vi "Actor Core.vi"(8 "error in (no error)":errorcluster, 11 "Operator UI.lvclass":refnum<class "Server UI.lvclass">) -> (0 "error out":errorcluster, 3 "Actor Framework.lvlib:Actor":refnum<class "Actor.lvclass">)   [LabVIEW 2026, in "Server UI.lvlib" / "Server UI.lvclass"]
doc: "This is Actor Core.vi, the main message handling loop for Actors. An actor usually just sits in this loop and processes messages as they arrive. Any error returned by the message Do.vi call will stop the loop, with error code 43 as the cannonical signal to stop with no error sent to caller. Descendants may override that in Handle Error.vi."
uses:
  Server UI.lvclass
  <vilib>/ActorFramework/Actor/Actor.lvclass
  Server UI.lvclass/Server UI.ctl
  <vilib>/ActorFramework/Actor/Actor.lvclass/Actor.ctl
  <vilib>/ActorFramework/Message Enqueuer/Message Enqueuer.lvclass/Message Enqueuer.ctl
  Write Start Server.vi
  Write Connected Clients.vi
  <vilib>/ActorFramework/Message Enqueuer/Init from Existing Queue.vi
  <vilib>/ActorFramework/Message Enqueuer/Enqueue.vi
  <vilib>/ActorFramework/Stop Msg/Stop Msg.lvclass
  MAL-Framework/user.lib/Common Components/User Interface/Messages/Disable UI Msg/Disable UI Msg.lvclass
  Server UI Messages/Show Connections Msg/Show Connections Msg.lvclass
  framework/Msmt UI/Messages/Ask Controller to Launch Results UI Msg/Ask Controller to Launch Results UI Msg.lvclass
  MAL-Framework/user.lib/Common Components/User Interface/Messages/Reset Controls Msg/Reset Controls Msg.lvclass
  Server UI Messages/Reset Measurement List Display Msg/Reset Measurement List Display Msg.lvclass
  framework/Measurement UI Messages/Launch Step Configuration Msg/Launch Step Configuration Msg.lvclass
  framework/User Interface/Messages/Enable UI Msg/Enable UI Msg.lvclass
  MAL-Framework/user.lib/Common Components/Msmt UI/Messages/Tell Controller to Launch Settings Dialog Msg/Tell Controller to Launch Settings Dialog Msg.lvclass
  framework/Msmt UI/Accessors/Write Digitizer.vi
  framework/Msmt UI/Accessors/Write Function Generator.vi
  framework/Msmt UI/Accessors/Write Load New Measurement.vi
  framework/Msmt UI/Accessors/Write Measurement.vi
  framework/Msmt UI/Accessors/Write Multimeter.vi
  framework/Msmt UI/Accessors/Write Power Supply.vi
  framework/Msmt UI/Accessors/Write Results Listbox.vi
  framework/Msmt UI/Accessors/Write Run.vi
  framework/Msmt UI/Accessors/Write Show FP_.vi
  framework/Msmt UI/Accessors/Write Status Display.vi
  framework/Msmt UI/Accessors/Write Tab Control.vi
  framework/Msmt UI/Accessors/Write View Results.vi
  framework/User Interface/Accessors/Write Settings Button.vi
  framework/Msmt UI/Write settings button array for hardware.vi
  framework/Msmt UI/Accessors/Write Step Config.vi
  <vilib>/ActorFramework/Message Priority Queue/Priority Enqueue.vi
  <vilib>/ActorFramework/Message Enqueuer/Message Enqueuer.lvclass
  framework/Msmt UI/Measurement UI.lvclass
  framework/Msmt UI/Messages/Send Run Measurement Message/Send Run Measurement Message.lvclass
  framework/Msmt UI/Messages/Send Get Hardware Info Message/Send Get Hardware Info Message.lvclass
  framework/Msmt UI/Messages/Check Run Button/Check Validity of Selection.lvclass
  framework/Msmt UI/Messages/Prompt User for Path to load/Prompt User for File Path to Load From.lvclass
  framework/User Interface/UI.lvclass
  framework/Measurement UI Messages/Launch Hardware Settings Msg/Launch Hardware Settings Msg.lvclass
panel:
  in  "Connected Clients":i32(listbox)
  in  "Step Config":bool
  in  "3":bool
  in  "2":bool
  in  "1":bool
  in  "0":bool
  in  "Show FP?":bool
  in  "Power Supply":u16(ring) caption="4"
  in  "Function Generator":u16(ring) caption="3"
  in  "Digitizer":u16(ring) caption="2"
  in  "Multimeter":u16(ring) caption="1"
  in  "Step":u16(ring)
  in  "about":bool
  in  "Tab Control":enum32{"Test Status", "Results"}(tab)
  in  "Status Display":string
  in  "View Results":bool
  in  "Results Listbox":i32(listbox)
  in  "Settings Button":bool
  in  "Start Server":bool
  in  "Load New Measurement":bool
  in  "Run":bool
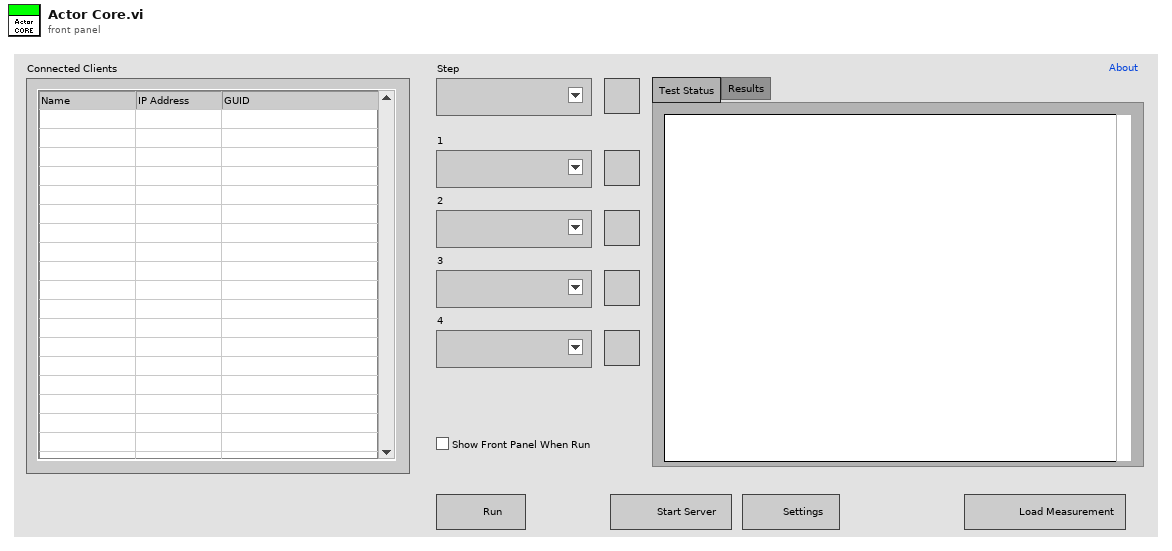
[diagram p1: front panel]
types:
  T1 = enum8{"Enabled", "Disabled", "Disabled and Grayed Out"}
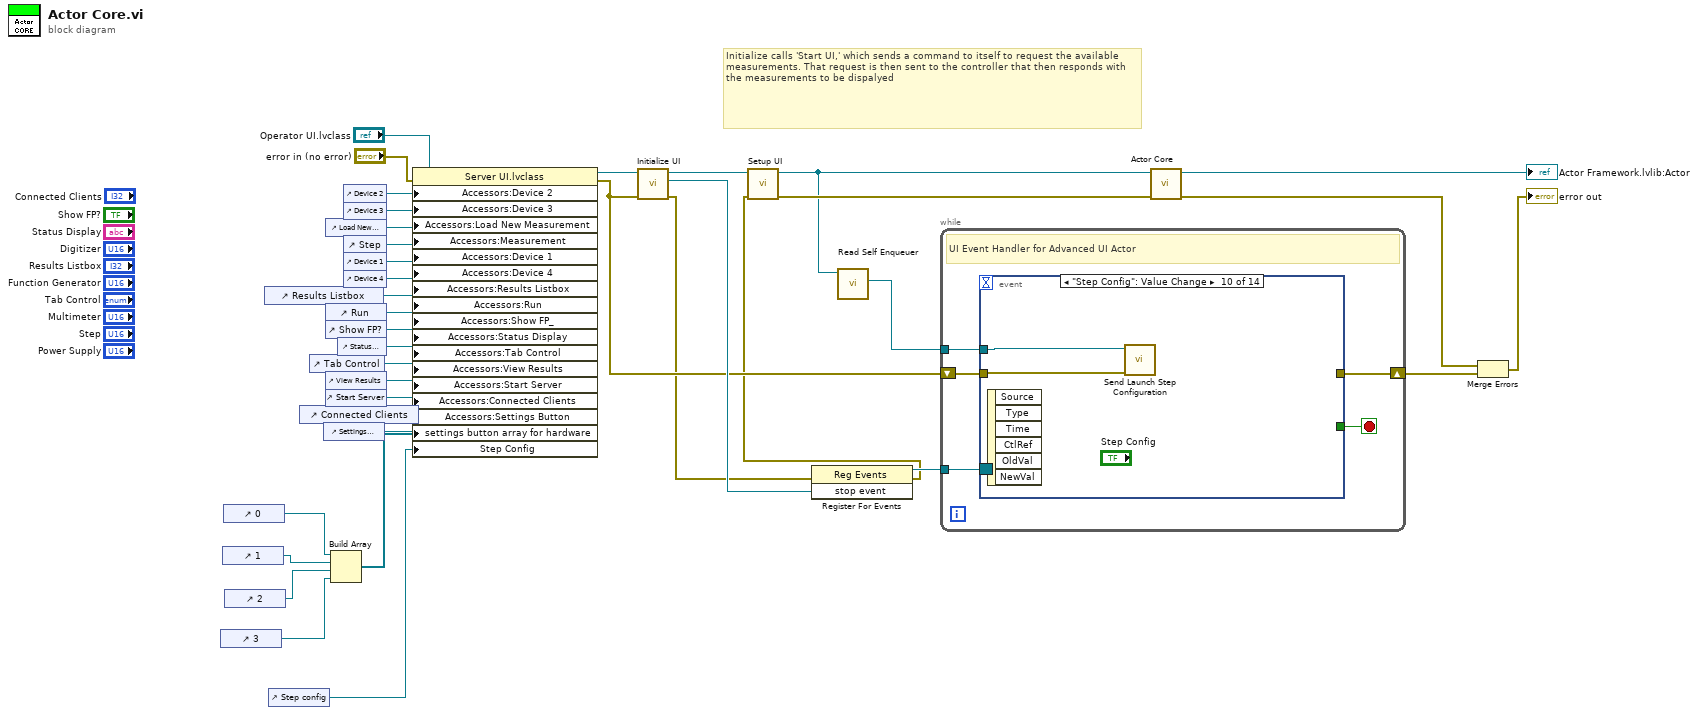
[diagram p0: block diagram]
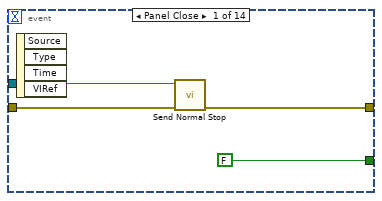
[diagram p2: hidden frame]
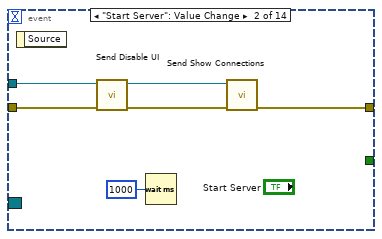
[diagram p3: hidden frame]
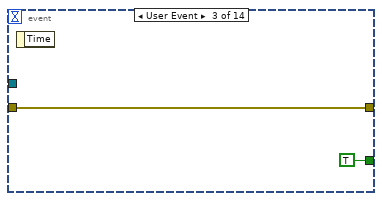
[diagram p4: hidden frame]
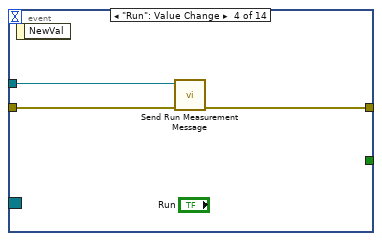
[diagram p5: hidden frame]
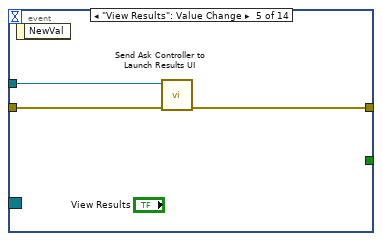
[diagram p6: hidden frame]
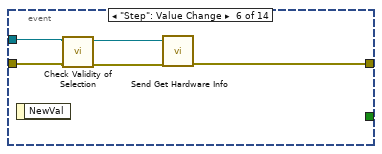
[diagram p7: hidden frame]
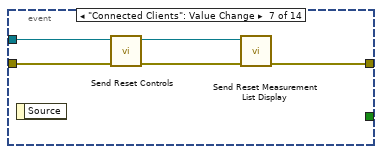
[diagram p8: hidden frame]
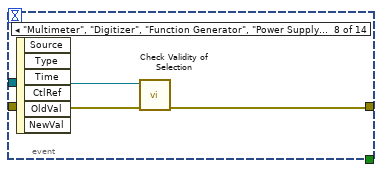
[diagram p9: hidden frame]
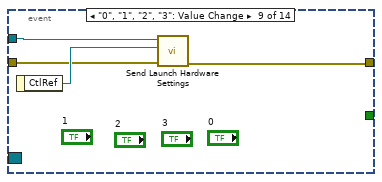
[diagram p10: hidden frame]
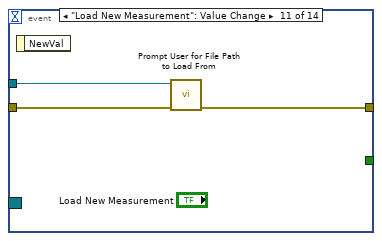
[diagram p11: hidden frame]
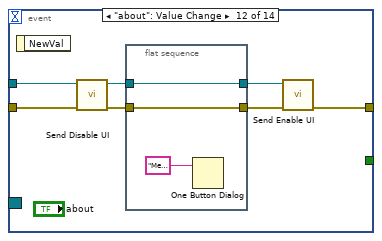
[diagram p12: hidden frame]
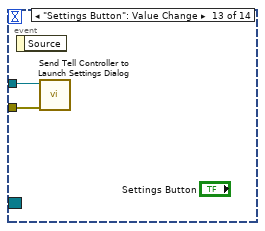
[diagram p13: hidden frame]
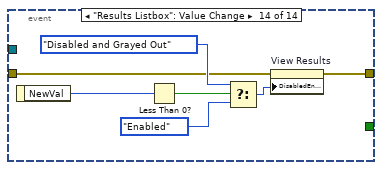
[diagram p14: hidden frame]
diagram:
  # "Initialize calls 'Start UI,' which sends a command to itself to request the available measurements. That request is then sent to the controller that then responds with the measurements to be dispalyed"
  n1 = control-ref of="3"() -> (w8:refnum<vi>)
  n2 = control-ref of="1"() -> (w6:refnum<vi>)
  n3 = control-ref of="0"() -> (w5:refnum<vi>)
  n4 = control-ref of="2"() -> (w7:refnum<vi>)
  n5 = control-ref of="Results Listbox"() -> (w28:refnum<vi>)
  n6 = control-ref of="Step config"() -> (w3:refnum<vi>)
  n7 = control-ref of="Connected Clients"() -> (w11:refnum<vi>)
  n8 = control-ref of="Tab Control"() -> (w30:refnum<vi>)
  n9 = control-ref of="Settings Button"() -> (w9:refnum<vi>)
  n10 = control-ref of="Load New Measurement"() -> (w24:refnum<vi>)
  n11 = control-ref of="Run"() -> (w21:refnum<vi>)
  n12 = control-ref of="Show FP?"() -> (w32:refnum<vi>)
  n13 = control-ref of="View Results"() -> (w29:refnum<vi>)
  n14 = control-ref of="Start Server"() -> (w12:refnum<vi>)
  n15 = Build Array(w5, w6, w7, w8) -> (w4:refnum<vi>[])
  n16 = control-ref of="Status Display"() -> (w31:refnum<vi>)
  n17 = control-ref of="Device 2"() -> (w26:refnum<vi>)
  n18 = control-ref of="Device 3"() -> (w25:refnum<vi>)
  n19 = control-ref of="Step"() -> (w23:refnum<vi>)
  n20 = control-ref of="Device 1"() -> (w22:refnum<vi>)
  n21 = control-ref of="Device 4"() -> (w27:refnum<vi>)
  n22 = property class="Server UI.lvclass"(reference="Operator UI.lvclass", error in="error in (no error)", "Accessors:Device 2"=w26, "Accessors:Device 3"=w25, "Accessors:Load New Measurement"=w24, "Accessors:Measurement"=w23, "Accessors:Device 1"=w22, "Accessors:Device 4"=w27, "Accessors:Results Listbox"=w28, "Accessors:Run"=w21, "Accessors:Show FP_"=w32, "Accessors:Status Display"=w31, "Accessors:Tab Control"=w30, "Accessors:View Results"=w29, "Accessors:Start Server"=w12, "Accessors:Connected Clients"=w11, "Accessors:Settings Button"=w9, "settings button array for hardware"=w4, "Step Config"=w3) -> (reference out=w16:refnum<class "Server UI.lvclass">, error out=w13:errorcluster)
  n23 = call "Initialize UI.vi"("error in (no error)"=w13, "UI in"=w16) -> ("error out"=w2:errorcluster, "stop event"=w33:refnum<user-event>, "UI out"=w15:refnum<class "Server UI.lvclass">)  [unwired: 7 in]
  n24 = register-events(error in=w2, w33) -> (reference out=w34:refnum<event-registration>, error out=w1:errorcluster)  [unwired: 1 in]
  n25 = call-dynamic "Setup UI.vi"("error in (no error)"=w1, "Operator UI in"=w15) -> ("error out"=w14:errorcluster, "Operator UI out"=w10:refnum<class "Server UI.lvclass">)  [unwired: 8 in]
  n26 = call <vilib>:"Read Self Enqueuer.vi"("Actor"=w10) -> ("Self Enqueuer"=w36:refnum<class "Message Enqueuer.lvclass">)  [unwired: 10 in]
  n27 = while {
    tunnel: w36 -> [w41]
    tunnel: w34 -> [w40]
    shift-right: [w38] -> w35
    shift-left: w13 -> [w39]
    stop <- w42 stop-if-true
    # "UI Event Handler for Advanced UI Actor"
    n28 = event shown="[9] \"Step Config\": Value Change" {
      selector: w40 -> [_ _ _ _ _ _ _ _ _ _ _ _ _ _]
      dyn-events: _ -> [_ _ _ _ _ _ _ _ _ _ _ _ _ _]
      timeout: _ -> [_ _ _ _ _ _ _ _ _ _ _ _ _ _]
      tunnel: [FALSE _ TRUE _ _ _ _ _ _ _ _ _ _ _] -> w42
      tunnel: w41 -> [w45 w50 _ w57 w60 w64 w70 w73 w77 w79 w82 w89 w93 _]
      tunnel: w39 -> [w44 w49 w53 w56 w59 w63 w69 w72 w75 w78 w81 w88 w94 w96]
      tunnel: [w43 w47 w53 w55 w58 w65 w66 w71 w74 _ w80 w83 _ w95] -> w38
      event Panel Close {
        n29 = event-data() -> ()  [unwired: 1 in, 4 out]
        n30 = call <vilib>:"Send Normal Stop.vi"("error in (no error)"=w44, "Message Enqueuer"=w45) -> ("error out"=w43:errorcluster)  [unwired: 9 in]
      }
      event "Start Server": Value Change {
        n31 = event-data() -> ()  [unwired: 1 in, 1 out]
        n32 = call "Send Disable UI.vi"("error in (no error)"=w49, "Message Enqueuer"=w50) -> ("error out"=w48:errorcluster, "Message Enqueuer out"=w51:refnum<class "Message Enqueuer.lvclass">)  [unwired: 8 in]
        n33 = Wait (ms)(milliseconds to wait=u32 1000) -> ()  [unwired: 1 out]
        n34 = call "Send Show Connections.vi"("error in (no error)"=w48, "Message Enqueuer"=w51) -> ("error out"=w47:errorcluster)  [unwired: 8 in, 1 out]
      }
      event User Event {
        n35 = event-data() -> ()  [unwired: 1 in, 1 out]
      }
      event "Run": Value Change {
        n36 = event-data() -> ()  [unwired: 1 in, 1 out]
        n37 = call "Send Run Measurement Message.vi"("error in (no error)"=w56, "Message Enqueuer in"=w57) -> ("error out"=w55:errorcluster)  [unwired: 8 in, 1 out]
      }
      event "View Results": Value Change {
        n38 = event-data() -> ()  [unwired: 1 in, 1 out]
        n39 = call "Send Ask Controller to Launch Results UI.vi"("error in (no error)"=w59, "Message Enqueuer in"=w60) -> ("error out"=w58:errorcluster)  [unwired: 8 in, 1 out]
      }
      event "Step": Value Change {
        n40 = event-data() -> ()  [unwired: 1 in, 1 out]
        n41 = call "Check Validity of Selection.vi"("error in (no error)"=w63, "Message Enqueuer in"=w64) -> ("error out"=w62:errorcluster, "Message Enqueuer out"=w61:refnum<class "Message Enqueuer.lvclass">)  [unwired: 8 in]
        n42 = call "Send Get Hardware Info.vi"("error in (no error)"=w62, "Message Enqueuer in"=w61) -> ("error out"=w65:errorcluster)  [unwired: 8 in, 1 out]
      }
      event "Connected Clients": Value Change {
        n43 = event-data() -> ()  [unwired: 1 in, 1 out]
        n44 = call "Send Reset Controls.vi"("error in (no error)"=w69, "Message Enqueuer"=w70) -> ("error out"=w67:errorcluster, "Message Enqueuer out"=w68:refnum<class "Message Enqueuer.lvclass">)  [unwired: 8 in]
        n45 = call "Send Reset Measurement List Display.vi"("error in (no error)"=w67, "Message Enqueuer"=w68) -> ("error out"=w66:errorcluster)  [unwired: 8 in, 1 out]
      }
      event "Multimeter", "Digitizer", "Function Generator", "Power Supply": Value Change {
        n46 = event-data() -> ()  [unwired: 1 in, 6 out]
        n47 = call "Check Validity of Selection.vi"("error in (no error)"=w72, "Message Enqueuer in"=w73) -> ("error out"=w71:errorcluster)  [unwired: 8 in, 1 out]
      }
      event "0", "1", "2", "3": Value Change {
        n48 = event-data() -> ("CtlRef"=w76:refnum<vi>)  [unwired: 1 in]
        n49 = call "Send Launch Hardware Settings.vi"("error in (no error)"=w75, "button ref"=w76, "Message Enqueuer"=w77) -> ("error out"=w74:errorcluster)  [unwired: 7 in, 1 out]
      }
      event "Step Config": Value Change {
        n50 = event-data() -> ()  [unwired: 1 in, 6 out]
        n51 = call "Send Launch Step Configuration.vi"("error in (no error)"=w78, "Message Enqueuer"=w79) -> ()  [unwired: 8 in, 2 out]
      }
      event "Load New Measurement": Value Change {
        n52 = event-data() -> ()  [unwired: 1 in, 1 out]
        n53 = call "Prompt User for File Path to Load From.vi"("error in (no error)"=w81, "Message Enqueuer in"=w82) -> ("error out"=w80:errorcluster)  [unwired: 8 in, 1 out]
      }
      event "about": Value Change {
        n54 = event-data() -> ()  [unwired: 1 in, 1 out]
        n55 = call "Send Disable UI.vi"("error in (no error)"=w88, "Message Enqueuer"=w89) -> ("error out"=w87:errorcluster, "Message Enqueuer out"=w85:refnum<class "Message Enqueuer.lvclass">)  [unwired: 8 in]
        n56 = flat-sequence {
          tunnel: [w91] -> w86
          tunnel: w87 -> [w91]
          tunnel: [w90] -> w84
          tunnel: w85 -> [w90]
          frame #0 {
            n57 = One Button Dialog(message="Measurement Manager v3.0 ALPHA RELEASE\n\nNational Instruments (C) 2013\nWritten in NI LabVIEW 2013 by Elijah Kerry \nElijah.Kerry@ni.com\n\nekerry.wordpress.com\nLatest version: bit.ly/lv_oomal") -> ()  [unwired: 1 in, 1 out]
          }
        }
        n58 = call "Send Enable UI.vi"("error in (no error)"=w86, "Message Enqueuer"=w84) -> ("error out"=w83:errorcluster)  [unwired: 8 in, 1 out]
      }
      event "Settings Button": Value Change {
        n59 = event-data() -> ()  [unwired: 1 in, 1 out]
        n60 = call "Send Tell Controller to Launch Settings Dialog.vi"("error in (no error)"=w94, "Message Enqueuer"=w93) -> ()  [unwired: 8 in, 2 out]
      }
      event "Results Listbox": Value Change {
        n61 = event-data() -> ("NewVal"=w97:i32)  [unwired: 1 in]
        n62 = Less Than 0?(x=w97) -> (x < 0?=w98:bool)
        n63 = Select(t=T1."Disabled and Grayed Out" ("Disabled"), s=w98, f=T1."Enabled" ("Disabled")) -> (s? t:f=w101:T1)
        n64 = property on="View Results" class="Bool"(error in=w96, "DisabledEnum"=w101) -> (error out=w95:errorcluster)  [unwired: 1 in, 1 out]
      }
    }
  }
  n65 = call-parent "Actor Core.vi"("error in (no error)"=w14, "Operator UI.lvclass"=w10) -> ("error out"=w19:errorcluster, "Actor Framework.lvlib:Actor"=→"Actor Framework.lvlib:Actor":refnum<class "Actor.lvclass">)  [unwired: 8 in]
  n66 = Merge Errors(w19, w35) -> (→"error out":errorcluster)
